vi "ConfigMultiPoint.vi"(8 "error in (no error)":errorcluster, 11 "HP3458aDMM in":refnum<class "HP3458aDMM.lvclass">) -> (0 "error out":errorcluster, 3 "HP3458aDMM out":refnum<class "HP3458aDMM.lvclass">)   [LabVIEW 2014, in "SamplerPlugins.lvlib" / "HP3458aDMM.lvclass"]
uses:
  HP3458aDMM.lvclass
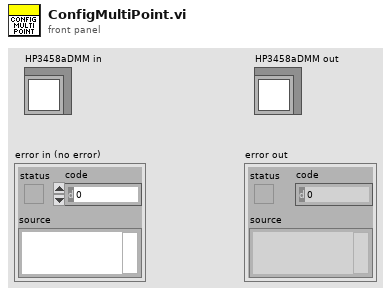
[diagram p1: front panel]
types:
  T1 = typedef "SamplerPlugins.lvlib/SamplerPluginsBase.lvclass/ConfigMultiPointParams.ctl" = cluster{"iTriggerCount":i32, "iSampleCount":i32, "eSampleClock":u16, "dSampleInterval":dbl}
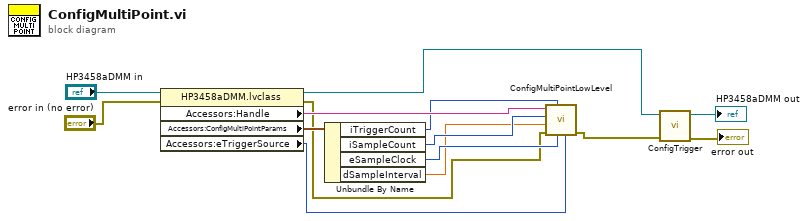
[diagram p0: block diagram]
diagram:
  n1 = property class="HP3458aDMM.lvclass"(reference="HP3458aDMM in", error in="error in (no error)") -> (reference out=w4:refnum<class "HP3458aDMM.lvclass">, error out=w6:errorcluster, "Accessors:Handle"=w11:string, "Accessors:ConfigMultiPointParams"=w12:T1, "Accessors:eTriggerSource"=w5:u16)
  n2 = Unbundle By Name(w12) -> ("iTriggerCount"=w10:i32, "iSampleCount"=w9:i32, "eSampleClock"=w8:u16, "dSampleInterval"=w7:dbl)
  n3 = call "ConfigMultiPointLowLevel.vi"("eTriggerSource"=w5, "eSampleTrigger"=w8, "iTriggerCount"=w10, "error in (no error)"=w6, "dSampleInterval"=w7, "iSampleCount"=w9, "HP3458 VISA resource name"=w11) -> ("error out"=w2:errorcluster)  [unwired: 4 in]
  n4 = call-dynamic "ConfigTrigger.vi"("error in (no error)"=w2, "HP3458aDMM in"=w4) -> ("error out"=→"error out":errorcluster, "HP3458aDMM out"=→"HP3458aDMM out":refnum<class "HP3458aDMM.lvclass">)  [unwired: 8 in]
